vi "Build.vi"(8 "error in (no error)":errorcluster, 11 "Field Factory in":refnum<class "Field Factory.lvclass">) -> (0 "error out":errorcluster, 2 "Column":refnum<class "Column Interface.lvclass">, 3 "Field Factory out":refnum<class "Field Factory.lvclass">)   [LabVIEW 2020]
uses:
  Column Configuration/Composed Column Factory.lvclass
  Basic Fields/Field Configurations/Field Configuration Class/Field Configuration.lvclass
  Column/Composed Column.lvclass
  Ctrl Renum Value Source Class/Ctrl Refnum Value Source.lvclass
  Text Ring Ctrl Refnum Source/Text Ring Ctrl Refnum Source.lvclass
  FK Field/FK Field.lvclass
  Composed Field/Composed Field.lvclass
  Field Factory.lvclass
  C:/Users/User/Desktop/Raman Program/Database OOP/source/Database OOP/Column Libraries/Column Configuration/Composed Column Factory.lvclass
  C:/Users/User/Desktop/Raman Program/Database OOP/source/Database OOP/Column Libraries/Basic Columns/Column Configuration/Column Factory Parent Class/Column Factory.lvclass
  C:/Users/User/Desktop/Raman Program/Database OOP/source/Database OOP/Column Libraries/Field Factory/Field Factory.lvclass
  C:/Users/User/Desktop/Raman Program/Database OOP/source/Database OOP/Column Libraries/Composed Field/Composed Field.lvclass
  C:/Users/User/Desktop/Raman Program/Database OOP/source/Database OOP/Column Libraries/Column/Composed Column.lvclass
  C:/Users/User/Desktop/Raman Program/Database OOP/source/Database OOP/Column Libraries/Column Interface/Column Interface Class/Column Interface.lvclass
  C:/Users/User/Desktop/Raman Program/Database OOP/source/Database OOP/Column Libraries/Field Interfaces/Field Interface Class/Field Interface.lvclass
  C:/Users/User/Desktop/Raman Program/Database OOP/source/Database OOP/Column Libraries/FK Field/FK Field.lvclass
  C:/Users/User/Desktop/Raman Program/Database OOP/source/Database OOP/Column Libraries/Ctrl Renum Value Source Class/Ctrl Refnum Value Source.lvclass
  C:/Users/User/Desktop/Raman Program/Database OOP/source/Database OOP/Column Libraries/Reference Value Source/Reference Value Source.lvclass
  C:/Users/User/Desktop/Raman Program/Database OOP/source/Database OOP/Column Libraries/Composed Columns/Value Source Interface Class/Value Source.lvclass
  C:/Users/User/Desktop/Raman Program/Database OOP/source/Database OOP/Column Libraries/Ring Ctrl Value Source/Ring Ctrl Value Source.lvclass
  C:/Users/User/Desktop/Raman Program/Database OOP/source/Database OOP/Column Libraries/Text Ring Ctrl Refnum Source/Text Ring Ctrl Refnum Source.lvclass
  Column Interface/Column Interface Class/Column Interface.lvclass
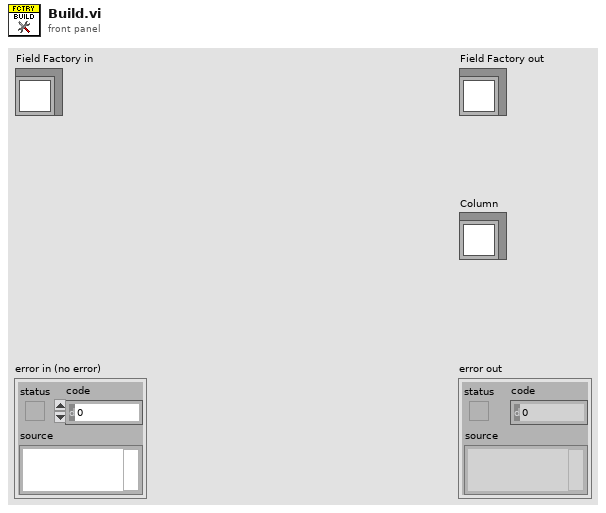
[diagram p1: front panel]
types:
  T1 = typedef "Column Interfaces.lvlib/FK Info.ctl" = cluster{"PK Table":string, "PK Column":string, "PK Display Column":string}
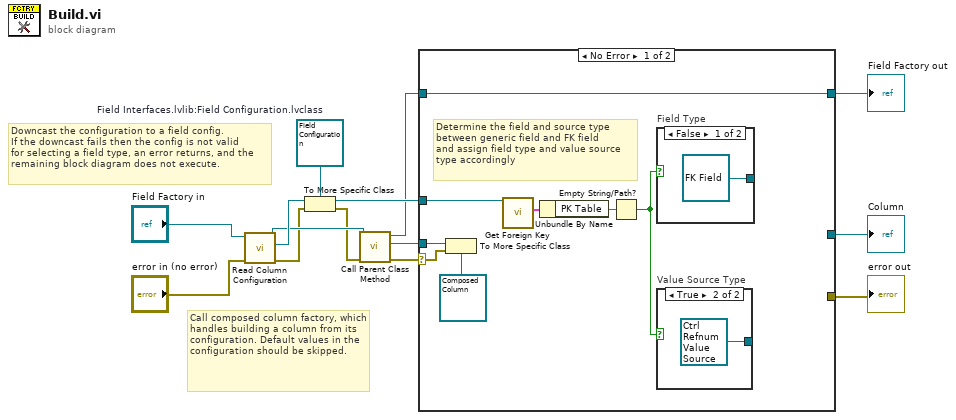
[diagram p0: block diagram]
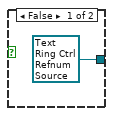
[diagram p2: hidden frame]
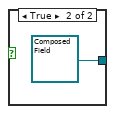
[diagram p3: hidden frame]
diagram:
  w12 = refnum<class "Field Configuration.lvclass"> refnum  # Field Interfaces.lvlib:Field Configuration.lvclass
  # "Call composed column factory, which handles building a column from its configuration. Default values in the configuration should be skipped."
  # "Downcast the configuration to a field config.\nIf the downcast fails then the config is not valid\nfor selecting a field type, an error returns, and the\nremaining block diagram does not execute."
  n1 = call "Read Column Configuration.vi"("error in (no error)"="error in (no error)", "Composed Column Factory in"="Field Factory in") -> ("error out"=w7:errorcluster, "Column Interfaces.lvlib:Column Configuration.lvclass"=w11:refnum<class "Column Configuration.lvclass">, "Composed Column Factory out"=w8:refnum<class "Field Factory.lvclass">)  [unwired: 7 in]
  n2 = To More Specific Class(target class=w12, reference=w11, error in=w7) -> (specific class reference=w10:refnum<class "Field Configuration.lvclass">, error out=w6:errorcluster)
  n3 = call-parent "Call Parent Class Method"("error in (no error)"=w6, "Composed Column Factory in"=w8) -> ("error out"=w3:errorcluster, "Column"=w2:refnum<class "Column Interface.lvclass">, "Composed Column Factory out"=w1:refnum<class "Field Factory.lvclass">)  [unwired: 7 in]
  n4 = case shown="No Error" w3 {
    selector: w3 -> [w19 w27]
    tunnel: w1 -> [w22 w29]
    tunnel: [w22 w29] -> w14
    tunnel: w2 -> [w21 w28]
    tunnel: [_ w28] -> w13
    tunnel: w10 -> [w18 _]
    tunnel: [_ w27] -> w9
    frame No Error {
      # "Determine the field and source type\nbetween generic field and FK field\nand assign field type and value source\ntype accordingly"
      n5 = To More Specific Class(target class=refnum<class "Composed Column.lvclass"> refnum ("Composed Columns.lvlib:Composed Column.lvclass"), reference=w21, error in=w19) -> ()  [unwired: 2 out]
      n6 = call-dynamic "Get Foreign Key.vi"("Basic Column Configuration in"=w18) -> ("FK Info"=w17:T1)  [unwired: 8 in, 2 out]
      n7 = Unbundle By Name(w17) -> ("PK Table"=w16:string)
      n8 = Empty String/Path?(string/path=w16) -> (empty?=w15:bool)
      n9 = case "Field Type" shown="False" w15 {
        tunnel: [refnum<class "FK Field.lvclass"> refnum ("Composed Fields.lvlib:FK Field.lvclass") refnum<class "Composed Field.lvclass"> refnum ("Composed Fields.lvlib:Composed Field.lvclass")] -> _
        frame False {
        }
        frame True {
        }
      }
      n10 = case "Value Source Type" shown="True" w15 {
        tunnel: [refnum<class "Text Ring Ctrl Refnum Source.lvclass"> refnum ("Composed Columns.lvlib:Text Ring Ctrl Refnum Source.lvclass") refnum<class "Ctrl Refnum Value Source.lvclass"> refnum ("Composed Columns.lvlib:Ctrl Refnum Value Source.lvclass")] -> _
        frame False {
        }
        frame True {
        }
      }
    }
    frame Error {
    }
  }
  "error out" <- w9
  "Field Factory out" <- w14
  "Column" <- w13
